vi "FPGA Main Image Processing.vi"(9 "Ocurrences":T1) -> ()   [LabVIEW 2017]
doc: "The myRIO v1.1 FPGA Shipping Personality. This personality contains support for:\n- 2 Analog Input Interrupt channel\n- 4 Digital Input Interrupt channel\n- 1 Timer\n- 1 Accelerometer\n- 1 Button\n- 4 LED\n- 10 Analog Input channels with 1 Sample\n- 6 Analog Output channels with 1 Sample\n- 40 Digital I/O channels with 1 Sample\n- 2 I2C channels\n- 4 Encoder channels\n- 6 PWM channels\n- 2 SPI channels"
uses:
  Controls/Ocurrences.ctl
  Controls/Image Size.ctl
  <vilib>/rvi/Emulation/niFpgaGetClockAttributes.vi
  <vilib>/rvi/Emulation/niFpgaSctlEmulationGetInTimedLoop.vi
  <vilib>/rvi/Emulation/niFpgaEmulationReportErrorSimple.vi
  <vilib>/rvi/Emulation/niFpgaProcessEmulError.vi
  <vilib>/rvi/DataTransferAndStorage/Container/Common/niFpgaContainerGetUniqueNameForEmu.vi
  <vilib>/rvi/DataTransferAndStorage/Container/Common/niFpgaContainerSetEmuInfo.vi
  <vilib>/rvi/eio/common/nirviEmuReportErrorAndStop.vi
  <vilib>/rvi/Memory/Memory_Emulation/nirvimemoryFastEmulation.vi
  <vilib>/rvi/Memory/Memory_Emulation/nirvimemoryEmulation.vi
  <vilib>/rvi/Emulation/niFpgaEmulationIsFPGAContextNoSignature.vi
  <vilib>/rvi/errors/nirviReportUnexpectedCaseInternalError (U32).vi
  <vilib>/rvi/interface/RandomDataEmulation/niFpgaRandomDataHandleErrors.vi
  <vilib>/rvi/Emulation/niFpgaCriticalErrorInLSC.vi
  <vilib>/rvi/LocalResourceManager/LocalResourceManager.xnode
  <vilib>/rvi/DataTransferAndStorage/Container/XNode/niFpgaContainer.xnode
  <vilib>/rvi/interface/RandomDataEmulation/nirviRandomDataFpgaReadWriteTemplate.vi
panel:
  out "Write TO":bool
  out "Read TO":bool
  out "Pixel B Write":u32
  out "Pixel A Write":u32
  out "Last Processed Pixel?":bool
  out "Pixel":u32
  out "Processing iteration":i32=-1
  out "Current Colum Process":u32
  out "Current Row Process":u32
  in  "Timeout":i32=-1
  out "Current Colum Write":u32
  out "Current Row Write":u32
  out "Last Write Pixel?":bool
  out "Last Read Pixel?":bool
  out "Current Colum Read":u32
  out "Current Row Read":u32
  out "Pixel B Write":u32
  out "Pixel A Write":u32
  out "Pixel B Read":u32
  out "Pixel A Read":u32
  out "SYS.OCURRENCES.RDY":bool
  out "FPGA to RT iteration":i32=-1
  out "RT to FPGA iteration":i32=-1
  out "SYS.IMG_SIZE.RDY":bool
  out "Image size":u32
  out "SYS.RDY":bool
  # "Image Processing"
  # "System"
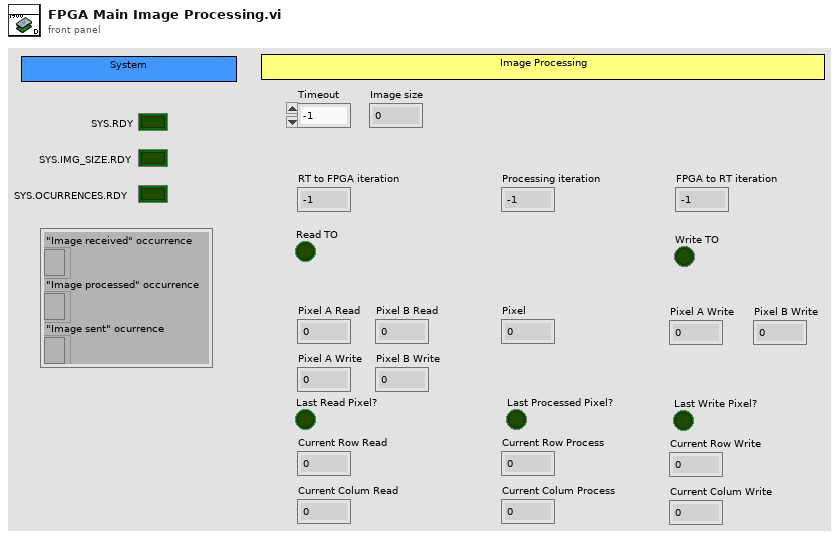
[diagram p1: front panel]
types:
  T1 = typedef "Ocurrences.ctl" = cluster{"\"Image received\" occurrence":refnum<k4>, "\"Image processed\" occurrence":refnum<k4>, "\"Image sent\" ocurrence":refnum<k4>}
  T2 = typedef "Image Size.ctl" = cluster{"Rows (X)":u16, "Colums (Y)":u16}
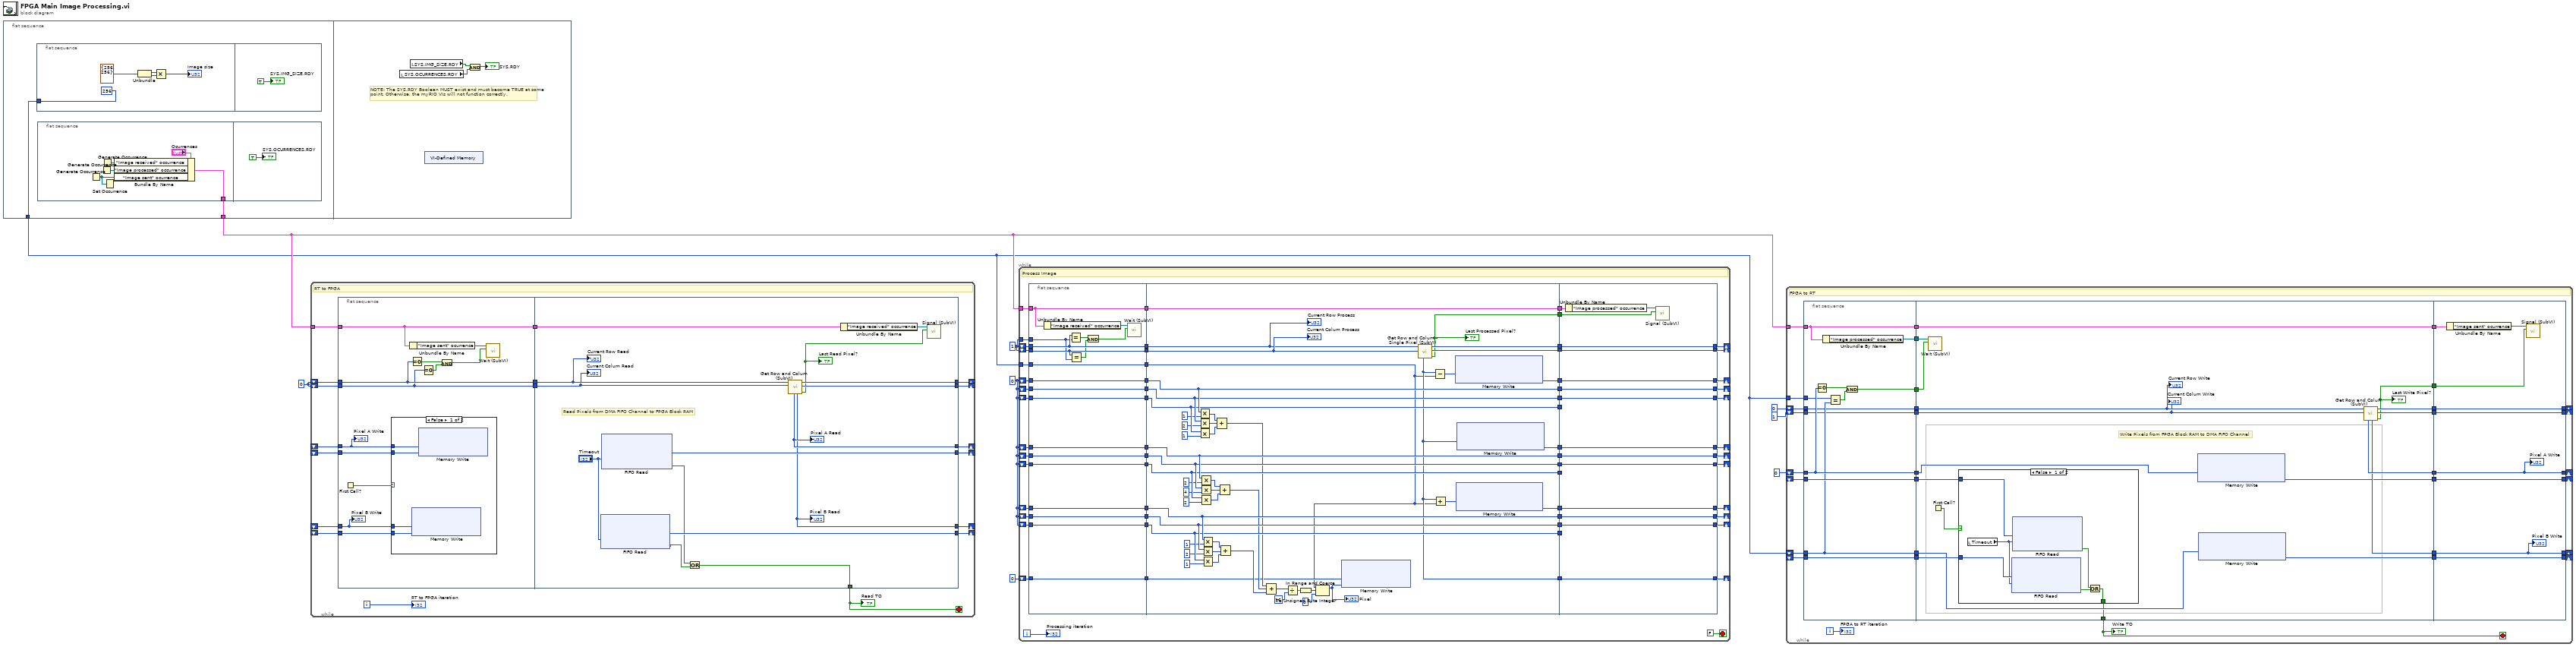
[diagram p0: block diagram]
diagram:
  w1 = u8 0 ("Data")
  w2 = u32 1 ("Row Out")
  w7 = u32 0
  n1 = flat-sequence {
    tunnel: [w11] -> w4
    tunnel: [w10] -> w5
    frame #0 {
      n2 = flat-sequence {
        tunnel: [u32 256 ("Dimension")] -> w11
        frame #0 {
          n3 = Unbundle(T2 {"Rows (X)"=256, "Colums (Y)"=256} ("Image Size")) -> ("Rows (X)"=w20:u16, "Colums (Y)"=w21:u16)
          n4 = Multiply(x=w20, y=w21) -> (x*y=→"Image size":u32)
        }
        frame #1 {
          "SYS.IMG_SIZE.RDY" <- TRUE
        }
      }
      n5 = flat-sequence {
        tunnel: [w12] -> w10
        frame #0 {
          n6 = Generate Occurrence() -> (w13:refnum<k4>)
          n7 = Generate Occurrence() -> (w14:refnum<k4>)
          n8 = Generate Occurrence() -> (w15:refnum<k4>)
          n9 = Set Occurrence(w13) -> ()
          n10 = Bundle By Name(cluster="Ocurrences", "\"Image received\" occurrence"=w15, "\"Image processed\" occurrence"=w14, "\"Image sent\" ocurrence"=w13) -> (w12:T1)
        }
        frame #1 {
          "SYS.OCURRENCES.RDY" <- TRUE
        }
      }
    }
    frame #1 {
      # "NOTE: The SYS.RDY Boolean MUST exist and must become TRUE at some point. Otherwise, the myRIO VIs will not function correctly."
      n11 = local read "SYS.OCURRENCES.RDY"() -> (w25:bool)
      n12 = local read "SYS.IMG_SIZE.RDY"() -> (w24:bool)
      n13 = xnode "VI-Defined Memory"() -> ()  [unwired: 1 out]
      n14 = And(x=w24, y=w25) -> (x .and. y?=→"SYS.RDY":bool)
    }
  }
  n15 = while {
    shift-right: [w36] -> _
    shift-left: _ -> [w43]
    shift-right: [w30] -> _
    shift-left: _ -> [w42]
    shift-right: [w35] -> _
    shift-left: _ -> [w41]
    shift-right: [w39] -> _
    shift-left: _ -> [w40]
    shift-right: [w38] -> _
    shift-left: w7 -> [w34]
    shift-right: [w37] -> _
    shift-left: w7 -> [w33]
    tunnel: w5 -> [w29]
    i -> [w44]
    stop <- w27 stop-if-true
    # "RT to FPGA"
    n16 = flat-sequence {
      tunnel: w33 -> [w54]
      tunnel: w34 -> [w55]
      tunnel: w40 -> [w47]
      tunnel: w41 -> [w45]
      tunnel: w42 -> [w48]
      tunnel: w43 -> [w46]
      tunnel: [w55] -> w32
      tunnel: [w54] -> w31
      tunnel: w29 -> [w56]
      tunnel: [w56] -> w28
      tunnel: w32 -> [w71]
      tunnel: w31 -> [w70]
      tunnel: w28 -> [w67]
      tunnel: [w75] -> w30
      tunnel: [w74] -> w39
      tunnel: [w73] -> w38
      tunnel: [w72] -> w37
      tunnel: [w66] -> w36
      tunnel: [w65] -> w35
      tunnel: [w61] -> w27
      frame #0 {
        n17 = First Call?() -> (First Call?: T/F=w49:bool)
        n18 = case shown="False" w49 {
          tunnel: w46 -> [w60 _]
          tunnel: w48 -> [w59 _]
          tunnel: w47 -> [w58 _]
          tunnel: w45 -> [w57 _]
          frame False {
            n19 = xnode ("Memory Write")("Address"=w57, "Data"=w58) -> ()  [unwired: 1 in, 1 out]
            n20 = xnode ("Memory Write")("Address"=w60, "Data"=w59) -> ()  [unwired: 1 in, 1 out]
          }
          frame True {
          }
        }
        n21 = Unbundle By Name(w56) -> ("\"Image sent\" ocurrence"=w51:refnum<k4>)
        n22 = Equal To 0?(x=w55) -> (x = 0?=w52:bool)
        n23 = Equal To 0?(x=w54) -> (x = 0?=w50:bool)
        n24 = And(x=w52, y=w50) -> (x .and. y?=w53:bool)
        n25 = call "Wait (SubVI).vi"("Wait? (T)"=w53, "Occurrence in"=w51) -> ()  [unwired: 10 in]
        "Pixel A Write" <- w46
        "Pixel B Write" <- w45
      }
      frame #1 {
        # "Read Pixels from DMA FIFO Channel to FPGA Block RAM"
        n26 = xnode ("FIFO Read")("Timeout"="Timeout") -> ("Element"=w74:u8, "Timed Out?"=w62:bool)  [unwired: 1 in, 1 out]
        n27 = xnode ("FIFO Read")("Timeout"="Timeout") -> ("Element"=w75:u8, "Timed Out?"=w63:bool)  [unwired: 1 in, 1 out]
        n28 = Or(x=w63, y=w62) -> (x .or. y?=w61:bool)
        n29 = call "Get Row and Colum (SubVI).vi"("Colum In"=w70, "Row In"=w71) -> ("Last Pixel?"=w69:bool, "Colum Out"=w72:u32, "Row Out"=w73:u32, "Pixel B"=w65:u32, "Pixel A"=w66:u32)  [unwired: 5 in]
        "Last Read Pixel?" <- w69
        "Pixel A Read" <- w66
        "Pixel B Read" <- w65
        n30 = Unbundle By Name(w67) -> ("\"Image received\" occurrence"=w64:refnum<k4>)
        n31 = call "Signal (SubVI).vi"("Set? (T)"=w69, "Occurrence in"=w64) -> ()  [unwired: 10 in]
        "Current Row Read" <- w71
        "Current Colum Read" <- w70
      }
    }
    "RT to FPGA iteration" <- w44
    "Read TO" <- w27
  }
  n32 = while {
    tunnel: w5 -> [w134]
    shift-right: [w130] -> _
    shift-left: w1 -> [w128]
    shift-right: [w126] -> _
    shift-left: w1 -> [w125]
    shift-right: [w122] -> _
    shift-left: w1 -> [w120]
    shift-right: [w117] -> _
    shift-left: w1 -> [w115]
    shift-right: [w113] -> _
    shift-left: w1 -> [w111]
    shift-right: [w109] -> _
    shift-left: w1 -> [w107]
    shift-right: [w104] -> _
    shift-left: w1 -> [w103]
    shift-right: [w100] -> _
    shift-left: w1 -> [w99]
    shift-right: [w96] -> _
    shift-left: w1 -> [w94]
    shift-right: [w91] -> _
    shift-left: w2 -> [w86]
    shift-right: [w89] -> _
    shift-left: w2 -> [w87]
    tunnel: w4 -> [w84]
    shift-right: [w80] -> _
    shift-left: u32 0 ("Pixel") -> [w82]
    tunnel: w2 -> [w78]
    i -> [w76]
    stop <- FALSE stop-if-true
    # "Process Image"
    n33 = flat-sequence {
      tunnel: w134 -> [w153]
      tunnel: [w153] -> w132
      tunnel: [w152] -> w129
      tunnel: w128 -> [w152]
      tunnel: w125 -> [w151]
      tunnel: [w151] -> w124
      tunnel: [w150] -> w121
      tunnel: w120 -> [w150]
      tunnel: [w149] -> w116
      tunnel: w115 -> [w149]
      tunnel: [w148] -> w112
      tunnel: w111 -> [w148]
      tunnel: [w147] -> w108
      tunnel: w107 -> [w147]
      tunnel: w103 -> [w146]
      tunnel: [w146] -> w102
      tunnel: w99 -> [w145]
      tunnel: [w145] -> w98
      tunnel: [w144] -> w95
      tunnel: w94 -> [w144]
      tunnel: [w141] -> w88
      tunnel: w87 -> [w141]
      tunnel: w86 -> [w140]
      tunnel: [w140] -> w85
      tunnel: w84 -> [w143]
      tunnel: [w143] -> w83
      tunnel: w82 -> [w142]
      tunnel: [w142] -> w81
      tunnel: w78 -> [w139]
      tunnel: [w204] -> w133
      tunnel: w132 -> [w204]
      tunnel: [w203] -> w131
      tunnel: w129 -> [w200]
      tunnel: [w200] -> w127
      tunnel: w124 -> [w199]
      tunnel: [w199] -> w123
      tunnel: w121 -> [w198]
      tunnel: [w198] -> w119
      tunnel: [w202] -> w118
      tunnel: w116 -> [w197]
      tunnel: [w197] -> w114
      tunnel: w112 -> [w196]
      tunnel: [w196] -> w110
      tunnel: w108 -> [w195]
      tunnel: [w195] -> w106
      tunnel: [w201] -> w105
      tunnel: w102 -> [w194]
      tunnel: [w194] -> w101
      tunnel: w98 -> [w193]
      tunnel: [w193] -> w97
      tunnel: w95 -> [w192]
      tunnel: [w192] -> w93
      tunnel: [w170] -> w92
      tunnel: [w169] -> w90
      tunnel: w88 -> [w160]
      tunnel: w85 -> [w161]
      tunnel: w83 -> [w162]
      tunnel: w81 -> [w166]
      tunnel: [w165] -> w79
      tunnel: [w159] -> w77
      tunnel: w133 -> [w219]
      tunnel: w131 -> [w217]
      tunnel: [w217] -> w130
      tunnel: w127 -> [w216]
      tunnel: [w216] -> w126
      tunnel: w123 -> [w215]
      tunnel: [w215] -> w122
      tunnel: w119 -> [_]
      tunnel: w118 -> [w214]
      tunnel: [w214] -> w117
      tunnel: w114 -> [w213]
      tunnel: [w213] -> w113
      tunnel: w110 -> [w212]
      tunnel: [w212] -> w109
      tunnel: w106 -> [_]
      tunnel: w105 -> [w211]
      tunnel: [w211] -> w104
      tunnel: w101 -> [w210]
      tunnel: [w210] -> w100
      tunnel: w97 -> [w209]
      tunnel: [w209] -> w96
      tunnel: w93 -> [_]
      tunnel: [w208] -> w91
      tunnel: w92 -> [w208]
      tunnel: w90 -> [w207]
      tunnel: [w207] -> w89
      tunnel: [w206] -> w80
      tunnel: w79 -> [w206]
      tunnel: w77 -> [w205]
      frame #0 {
        n34 = Unbundle By Name(w153) -> ("\"Image received\" occurrence"=w154:refnum<k4>)
        n35 = Equal?(x=w141, y=w139) -> (x = y?=w138:bool)
        n36 = Equal?(x=w140, y=w139) -> (x = y?=w137:bool)
        n37 = And(x=w138, y=w137) -> (x .and. y?=w136:bool)
        n38 = call "Wait (SubVI).vi"("Wait? (T)"=w136, "Occurrence in"=w154) -> ()  [unwired: 10 in]
      }
      frame #1 {
        n39 = Multiply(x=w200, y=i16 1) -> (x*y=w186:i16)
        n40 = Multiply(x=w199, y=i16 2) -> (x*y=w188:i16)
        n41 = Multiply(x=w198, y=i16 1) -> (x*y=w187:i16)
        n42 = Multiply(x=w197, y=i16 2) -> (x*y=w185:i16)
        n43 = Multiply(x=w196, y=i16 4) -> (x*y=w184:i16)
        n44 = Multiply(x=w195, y=i16 2) -> (x*y=w183:i16)
        n45 = Multiply(x=w194, y=i16 1) -> (x*y=w191:i16)
        n46 = Multiply(x=w193, y=i16 2) -> (x*y=w190:i16)
        n47 = Multiply(x=w192, y=i16 1) -> (x*y=w189:i16)
        n48 = Compound Arithmetic op=ADD(w186, w188, w187) -> (w182:i16)
        n49 = Compound Arithmetic op=ADD(w185, w184, w183) -> (w181:i16)
        n50 = Compound Arithmetic op=ADD(w191, w190, w189) -> (w180:i16)
        n51 = Compound Arithmetic op=ADD(w182, w181, w180) -> (w158:i16)
        n52 = Divide(x=w158, y=i16 16) -> (x/y=w156:fxp<+,8,8>)
        n53 = To Unsigned Byte Integer(number=w156) -> (unsigned 8bit integer=w155:u8)
        n54 = In Range and Coerce(upper limit=w162, x=w155, lower limit=i16 0) -> (coerced(x)=w164:u32)  [unwired: 1 out]
        "Pixel" <- w164
        n55 = xnode ("Memory Write")("Address"=w166, "Data"=w164) -> ()  [unwired: 1 in, 1 out]
        n56 = call "Get Row and Colum - Single Pixel (SubVI).vi"("Colum In"=w161, "Row In"=w160) -> ("Last Pixel?"=w159:bool, "Colum Out"=w170:u32, "Row Out"=w169:u32, "Pixel"=w165:u32)  [unwired: 6 in]
        "Last Processed Pixel?" <- w159
        n57 = Subtract(x=w165, y=w162) -> (x-y=w167:u32)
        n58 = Add(x=w165, y=w162) -> (x+y=w168:u32)
        n59 = xnode ("Memory Write")("Address"=w167) -> ("Data"=w203:u8)  [unwired: 1 in, 1 out]
        n60 = xnode ("Memory Write")("Address"=w168) -> ("Data"=w201:u8)  [unwired: 1 in, 1 out]
        n61 = xnode ("Memory Write")("Address"=w165) -> ("Data"=w202:u8)  [unwired: 1 in, 1 out]
        "Current Row Process" <- w160
        "Current Colum Process" <- w161
      }
      frame #2 {
        n62 = Unbundle By Name(w219) -> ("\"Image processed\" occurrence"=w218:refnum<k4>)
        n63 = call "Signal (SubVI).vi"("Set? (T)"=w205, "Occurrence in"=w218) -> ()  [unwired: 10 in]
      }
    }
    "Processing iteration" <- w76
  }
  n64 = while {
    shift-right: [w248] -> _
    shift-left: u32 0 -> [w252]
    shift-right: [w247] -> _
    shift-left: w4 -> [w251]
    shift-right: [w250] -> _
    shift-left: u32 0 -> [w246]
    shift-right: [w249] -> _
    shift-left: u32 1 ("Colum Out") -> [w245]
    shift-right: [w235] -> _
    shift-left: _ -> [w231]
    shift-right: [w233] -> _
    shift-left: _ -> [w229]
    tunnel: w4 -> [w225]
    tunnel: w5 -> [w224]
    i -> [w237]
    stop <- w220 stop-if-true
    # "FPGA to RT"
    n65 = flat-sequence {
      tunnel: w245 -> [w256]
      tunnel: w246 -> [w257]
      tunnel: w251 -> [w259]
      tunnel: w252 -> [w260]
      tunnel: [w260] -> w244
      tunnel: [w259] -> w243
      tunnel: [w262] -> w232
      tunnel: w231 -> [w262]
      tunnel: [w261] -> w230
      tunnel: w229 -> [w261]
      tunnel: [w258] -> w228
      tunnel: [w257] -> w227
      tunnel: [w256] -> w226
      tunnel: w225 -> [w255]
      tunnel: w224 -> [w254]
      tunnel: [w254] -> w223
      tunnel: [w253] -> w221
      tunnel: w244 -> [w272]
      tunnel: w243 -> [w271]
      tunnel: [w282] -> w242
      tunnel: [w281] -> w241
      tunnel: [w280] -> w240
      tunnel: [w279] -> w239
      tunnel: [w278] -> w238
      tunnel: [w277] -> w236
      tunnel: [w276] -> w234
      tunnel: w232 -> [w275]
      tunnel: w230 -> [w274]
      tunnel: w228 -> [w268]
      tunnel: w227 -> [w270]
      tunnel: w226 -> [w269]
      tunnel: w223 -> [w267]
      tunnel: [w267] -> w222
      tunnel: w221 -> [w266]
      tunnel: [w265] -> w220
      tunnel: [w294] -> w247
      tunnel: [w295] -> w248
      tunnel: [w296] -> w249
      tunnel: [w297] -> w250
      tunnel: w242 -> [w297]
      tunnel: w241 -> [w296]
      tunnel: w240 -> [w295]
      tunnel: w239 -> [w294]
      tunnel: w238 -> [w291]
      tunnel: [w293] -> w235
      tunnel: w236 -> [w293]
      tunnel: [w292] -> w233
      tunnel: w234 -> [w292]
      tunnel: w222 -> [w290]
      frame #0 {
        n66 = Equal To 0?(x=w260) -> (x = 0?=w263:bool)
        n67 = Unbundle By Name(w254) -> ("\"Image processed\" occurrence"=w253:refnum<k4>)
        n68 = Equal?(x=w255, y=w259) -> (x = y?=w264:bool)
        n69 = And(x=w263, y=w264) -> (x .and. y?=w258:bool)
      }
      frame #1 {
        # "Write Pixels from FPGA Block RAM to DMA FIFO Channel"
        n70 = call "Wait (SubVI).vi"("Wait? (T)"=w268, "Occurrence in"=w266) -> ()  [unwired: 10 in]
        n71 = First Call?() -> (First Call?: T/F=w273:bool)
        n72 = case shown="False" w273 {
          tunnel: w275 -> [w288 _]
          tunnel: w274 -> [w287 _]
          tunnel: [w283 _] -> w265
          frame False {
            n73 = local read "Timeout"() -> (w286:i32)
            n74 = xnode ("FIFO Read")("Element"=w287, "Timeout"=w286) -> ("Timed Out?"=w285:bool)  [unwired: 1 in, 1 out]
            n75 = xnode ("FIFO Read")("Element"=w288, "Timeout"=w286) -> ("Timed Out?"=w284:bool)  [unwired: 1 in, 1 out]
            n76 = Or(x=w284, y=w285) -> (x .or. y?=w283:bool)
          }
          frame True {
          }
        }
        n77 = xnode ("Memory Write")("Address"=w272) -> ("Data"=w277:u8)  [unwired: 1 in, 1 out]
        n78 = xnode ("Memory Write")("Address"=w271) -> ("Data"=w276:u8)  [unwired: 1 in, 1 out]
        n79 = call "Get Row and Colum (SubVI).vi"("Colum In"=w269, "Row In"=w270) -> ("Last Pixel?"=w278:bool, "Colum Out"=w281:u32, "Row Out"=w282:u32, "Pixel B"=w279:u32, "Pixel A"=w280:u32)  [unwired: 5 in]
        "Last Write Pixel?" <- w278
        "Current Row Write" <- w270
        "Current Colum Write" <- w269
      }
      frame #2 {
        n80 = Unbundle By Name(w290) -> ("\"Image sent\" ocurrence"=w289:refnum<k4>)
        n81 = call "Signal (SubVI).vi"("Set? (T)"=w291, "Occurrence in"=w289) -> ()  [unwired: 10 in]
        "Pixel A Write" <- w295
        "Pixel B Write" <- w294
      }
    }
    "FPGA to RT iteration" <- w237
    "Write TO" <- w220
  }
